vi "Init Async View.vi"(8 "error in (no error)":errorcluster, 11 "base view in":refnum<class "base view.lvclass">) -> (0 "error out":errorcluster, 3 "base view out":refnum<class "base view.lvclass">)   [LabVIEW 2022 SP3, in "base view.lvclass"]
uses:
  base view.lvclass
  Accessors/Read View Refnum.vi
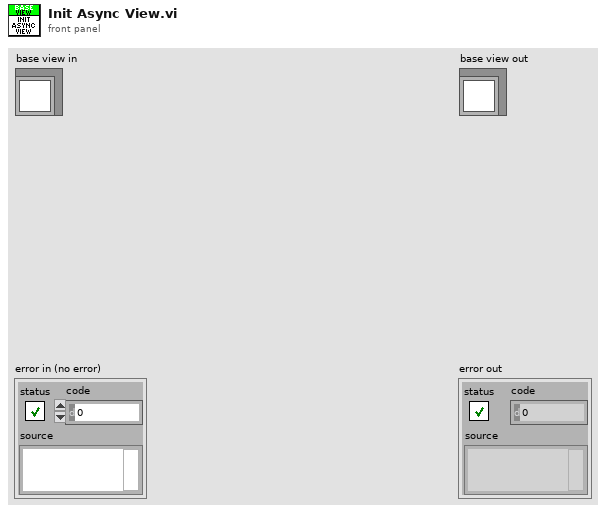
[diagram p1: front panel]
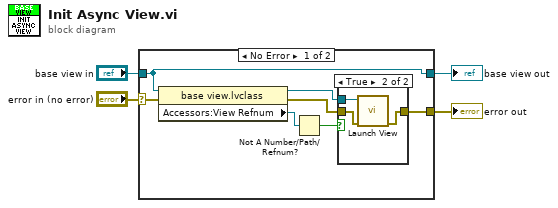
[diagram p0: block diagram]
diagram:
  n1 = case shown="No Error" "error in (no error)" {
    selector: "error in (no error)" -> [w6 w17]
    tunnel: [w5 w17] -> w3
    tunnel: [w11 w16] -> w1
    tunnel: "base view in" -> [w11 w16]
    frame No Error {
      n2 = property class="base view.lvclass"(reference=w11, error in=w6) -> (reference out=w8:refnum<class "base view.lvclass">, error out=w7:errorcluster, "Accessors:View Refnum"=w10:refnum<vi>)
      n3 = Not A Number/Path/Refnum?(number/path/refnum=w10) -> (NaN/Path/Refnum?=w9:bool)
      n4 = case shown="True" w9 {
        tunnel: w8 -> [_ w15]
        tunnel: w7 -> [w12 w14]
        tunnel: [w12 w13] -> w5
        frame False {
        }
        frame True {
          n5 = call "Launch View.vi"("error in (no error)"=w14, "base view in"=w15) -> ("error out"=w13:errorcluster)  [unwired: 8 in, 1 out]
        }
      }
    }
    frame Error {
    }
  }
  "error out" <- w3
  "base view out" <- w1
